vi "Handle after Disconnection.vi"(8 "error in (no error)":errorcluster, 11 "Connection In":refnum<k5>) -> (0 "error out":errorcluster, 3 "Connection out":refnum<k5>)   [LabVIEW 2015]
uses:
  Global/SeverGlobal.vi
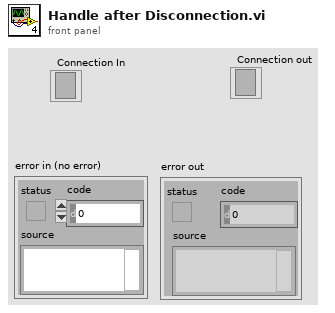
[diagram p1: front panel]
types:
  T1 = cluster{"TCP Ref":refnum<k5>, "Broadcast":refnum<k5>, "TF Ref":refnum<k5>, "IP":string, "port":u16, "userName":string, "passWord":string, "authority":string}[]
  T2 = cluster{"TCP Ref":refnum<k5>, "IP":string, "userName":string, "A":u16, "COM":u16, "time":u32}[]
  T3 = cluster{"TCP Ref":refnum<k5>, "IP":string, "userName":string, "IN":u16, "OUT":u16, "time":u32}[]
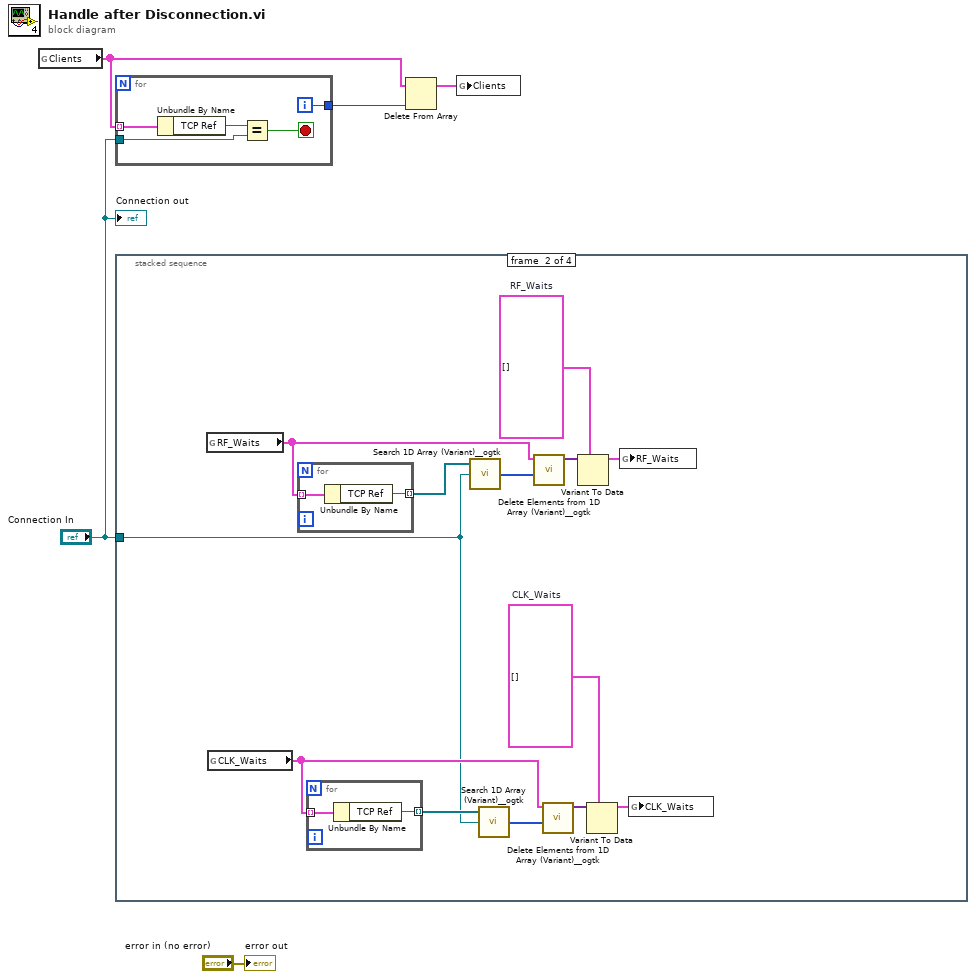
[diagram p0: block diagram]
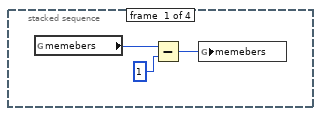
[diagram p2: hidden frame]
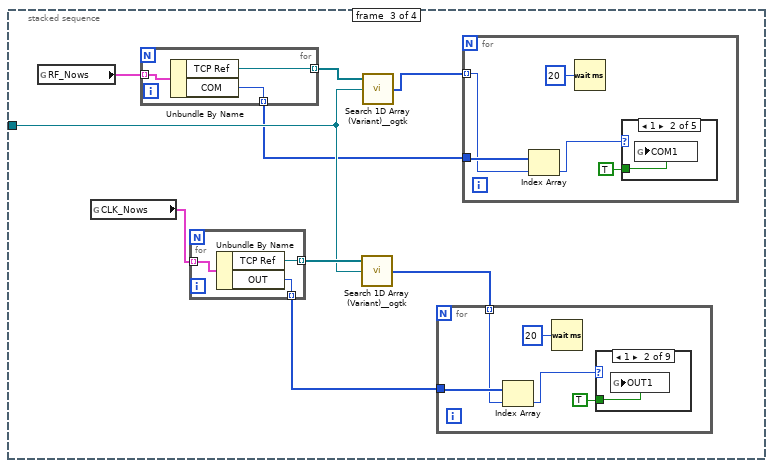
[diagram p3: hidden frame]
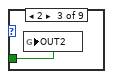
[diagram p5: hidden frame]
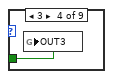
[diagram p6: hidden frame]
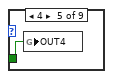
[diagram p7: hidden frame]
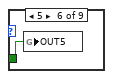
[diagram p8: hidden frame]
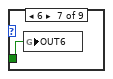
[diagram p9: hidden frame]
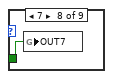
[diagram p10: hidden frame]
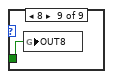
[diagram p11: hidden frame]
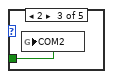
[diagram p13: hidden frame]
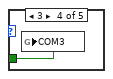
[diagram p14: hidden frame]
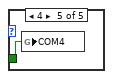
[diagram p15: hidden frame]
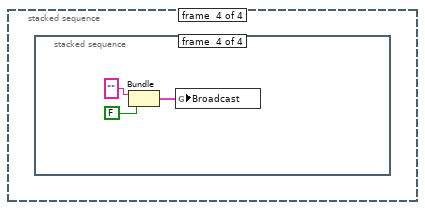
[diagram p16: hidden frame]
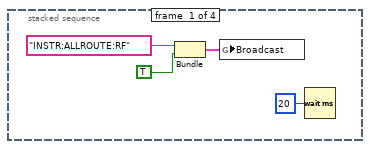
[diagram p17: hidden frame]
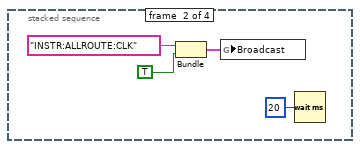
[diagram p18: hidden frame]
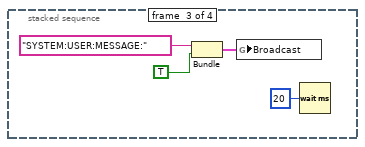
[diagram p19: hidden frame]
diagram:
  n1 = global read "SeverGlobal.vi" "Clients"() -> (w5:T1)
  n2 = for {
    tunnel: w5 -> [w10] mode=indexing
    tunnel: "Connection In" -> [w8]
    tunnel: [w6] -> w1
    i -> [w6]
    stop <- w7 stop-if-true
    n3 = Unbundle By Name(w10) -> ("TCP Ref"=w9:refnum<k5>)
    n4 = Equal?(x=w9, y=w8) -> (x = y?=w7:bool)
  }
  n5 = stacked-sequence {
    tunnel: "Connection In" -> [_ w14 w35 _]
    frame #0 {
      n6 = global read "SeverGlobal.vi" "memebers"() -> (w13:i32)
      n7 = Subtract(x=w13, y=1) -> (x-y=w11:i32)
      n8 = global write "SeverGlobal.vi" "memebers"(w11) -> ()
    }
    frame #1 {
      w16 = T2 []  # CLK_Waits
      w25 = T2 []  # RF_Waits
      n9 = global read "SeverGlobal.vi" "RF_Waits"() -> (w23:T2)
      n10 = global read "SeverGlobal.vi" "CLK_Waits"() -> (w18:T3)
      n11 = for {
        tunnel: w23 -> [w30] mode=indexing
        tunnel: [w29] -> w21 mode=indexing
        n12 = Unbundle By Name(w30) -> ("TCP Ref"=w29:refnum<k5>)
      }
      n13 = for {
        tunnel: w18 -> [w28] mode=indexing
        tunnel: [w27] -> w20 mode=indexing
        n14 = Unbundle By Name(w28) -> ("TCP Ref"=w27:refnum<k5>)
      }
      n15 = call <userlib>:"Search 1D Array (Variant)__ogtk.vi"("Array"=w21, "Element Data"=w14) -> ("Indices of Elements"=w22:i32[])  [unwired: 7 in]
      n16 = call <userlib>:"Search 1D Array (Variant)__ogtk.vi"("Array"=w20, "Element Data"=w14) -> ("Indices of Elements"=w19:i32[])  [unwired: 7 in]
      n17 = call <userlib>:"Delete Elements from 1D Array (Variant)__ogtk.vi"("indices"=w22, "array"=w23) -> ("array w/ subset deleted"=w24:variant[])  [unwired: 8 in, 1 out]
      n18 = call <userlib>:"Delete Elements from 1D Array (Variant)__ogtk.vi"("indices"=w19, "array"=w18) -> ("array w/ subset deleted"=w17:variant[])  [unwired: 8 in, 1 out]
      n19 = Variant To Data(type=w25, Variant=w24) -> (data=w26:T2)  [unwired: 1 in, 1 out]
      n20 = Variant To Data(type=w16, Variant=w17) -> (data=w15:T2)  [unwired: 1 in, 1 out]
      n21 = global write "SeverGlobal.vi" "RF_Waits"(w26) -> ()
      n22 = global write "SeverGlobal.vi" "CLK_Waits"(w15) -> ()
    }
    frame #2 {
      n23 = global read "SeverGlobal.vi" "RF_Nows"() -> (w39:T2)
      n24 = global read "SeverGlobal.vi" "CLK_Nows"() -> (w36:T3)
      n25 = for {
        tunnel: w39 -> [w67] mode=indexing
        tunnel: [w66] -> w38 mode=indexing
        tunnel: [w65] -> w34 mode=indexing
        n26 = Unbundle By Name(w67) -> ("TCP Ref"=w66:refnum<k5>, "COM"=w65:u16)
      }
      n27 = for {
        tunnel: w36 -> [w64] mode=indexing
        tunnel: [w63] -> w37 mode=indexing
        tunnel: [w62] -> w31 mode=indexing
        n28 = Unbundle By Name(w64) -> ("TCP Ref"=w63:refnum<k5>, "OUT"=w62:u16)
      }
      n29 = call <userlib>:"Search 1D Array (Variant)__ogtk.vi"("Array"=w37, "Element Data"=w35) -> ("Indices of Elements"=w32:i32[])  [unwired: 7 in]
      n30 = call <userlib>:"Search 1D Array (Variant)__ogtk.vi"("Array"=w38, "Element Data"=w35) -> ("Indices of Elements"=w33:i32[])  [unwired: 7 in]
      n31 = for {
        tunnel: w31 -> [w43]
        tunnel: w32 -> [w42] mode=indexing
        n32 = Index Array(array=w43, index=w42) -> (element=w41:u16)
        n33 = Wait (ms)(milliseconds to wait=u32 20) -> ()  [unwired: 1 out]
        n34 = case shown="1" w41 {
          tunnel: TRUE -> [_ w45 w46 w47 w48 w49 w50 w51 w52]
          frame 0, Default {
          }
          frame 1 {
            n35 = global write "SeverGlobal.vi" "OUT1"(w45) -> ()
          }
          frame 2 {
            n36 = global write "SeverGlobal.vi" "OUT2"(w46) -> ()
          }
          frame 3 {
            n37 = global write "SeverGlobal.vi" "OUT3"(w47) -> ()
          }
          frame 4 {
            n38 = global write "SeverGlobal.vi" "OUT4"(w48) -> ()
          }
          frame 5 {
            n39 = global write "SeverGlobal.vi" "OUT5"(w49) -> ()
          }
          frame 6 {
            n40 = global write "SeverGlobal.vi" "OUT6"(w50) -> ()
          }
          frame 7 {
            n41 = global write "SeverGlobal.vi" "OUT7"(w51) -> ()
          }
          frame 8 {
            n42 = global write "SeverGlobal.vi" "OUT8"(w52) -> ()
          }
        }
      }
      n43 = for {
        tunnel: w34 -> [w56]
        tunnel: w33 -> [w55] mode=indexing
        n44 = Index Array(array=w56, index=w55) -> (element=w54:u16)
        n45 = Wait (ms)(milliseconds to wait=u32 20) -> ()  [unwired: 1 out]
        n46 = case shown="1" w54 {
          tunnel: TRUE -> [_ w58 w59 w60 w61]
          frame 0, Default {
          }
          frame 1 {
            n47 = global write "SeverGlobal.vi" "COM1"(w58) -> ()
          }
          frame 2 {
            n48 = global write "SeverGlobal.vi" "COM2"(w59) -> ()
          }
          frame 3 {
            n49 = global write "SeverGlobal.vi" "COM3"(w60) -> ()
          }
          frame 4 {
            n50 = global write "SeverGlobal.vi" "COM4"(w61) -> ()
          }
        }
      }
    }
    frame #3 {
      n51 = stacked-sequence {
        frame #0 {
          n52 = Bundle("INSTR:ALLROUTE:RF", TRUE) -> (w69:cluster{string, bool})  [unwired: 1 in]
          n53 = global write "SeverGlobal.vi" "Broadcast"(w69) -> ()
          n54 = Wait (ms)(milliseconds to wait=u32 20) -> ()  [unwired: 1 out]
        }
        frame #1 {
          n55 = Bundle("INSTR:ALLROUTE:CLK", TRUE) -> (w73:cluster{string, bool})  [unwired: 1 in]
          n56 = global write "SeverGlobal.vi" "Broadcast"(w73) -> ()
          n57 = Wait (ms)(milliseconds to wait=u32 20) -> ()  [unwired: 1 out]
        }
        frame #2 {
          n58 = Bundle("SYSTEM:USER:MESSAGE:", TRUE) -> (w79:cluster{string, bool})  [unwired: 1 in]
          n59 = global write "SeverGlobal.vi" "Broadcast"(w79) -> ()
          n60 = Wait (ms)(milliseconds to wait=u32 20) -> ()  [unwired: 1 out]
        }
        frame #3 {
          n61 = Bundle("", FALSE) -> (w80:cluster{string, bool})  [unwired: 1 in]
          n62 = global write "SeverGlobal.vi" "Broadcast"(w80) -> ()
        }
      }
    }
  }
  n63 = Delete From Array(array=w5, index=w1) -> (array with subset deleted=w4:T1)  [unwired: 1 in, 1 out]
  n64 = global write "SeverGlobal.vi" "Clients"(w4) -> ()
  "error out" <- "error in (no error)"
  "Connection out" <- "Connection In"
